vi "Li_New_ADDR_svi.vi"(7 "Op":T1(ring), 8 "error in (no error)":errorcluster, 9 "Addr":i32, 10 "Name":string="FREE") -> (0 "error out":errorcluster, 2 "Size":i32, 3 "Addr":i32)   [LabVIEW 2015]
uses:
  index_cluster.ctl
  C:/Users/Giuseppe/Downloads/LabLinda_ pakage/index_datatype.ctl
  C:/Users/Giuseppe/Downloads/LabLinda_ pakage/index_cluster.ctl
  LIFO.ctl
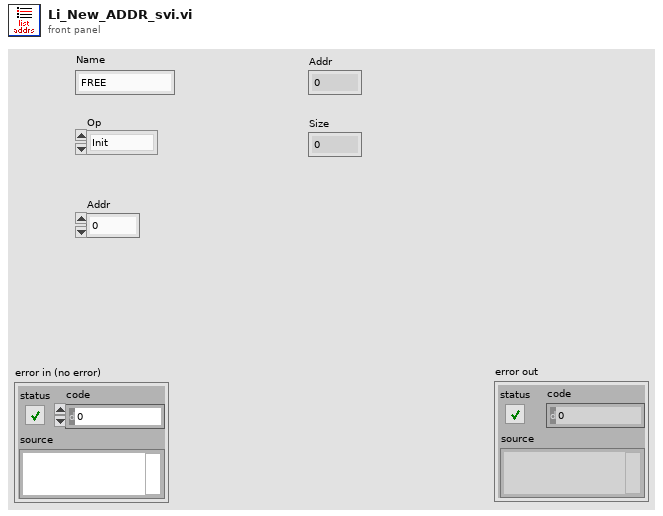
[diagram p1: front panel]
types:
  T1 = enum16{"Init", "Read addr", "Write item", "Cleanup", "Add free", "Query Free"}
  T2 = typedef "index_cluster.ctl" = cluster{"Addr":i32[], "out react vi reference":refnum<vi>, "in react vi reference":refnum<vi>, "rd react vi reference":refnum<vi>, "Read_write_var":refnum<vi>}
  T3 = typedef "LIFO.ctl" = enum16{"INIT", "Push", "Pop", "Query", "BPush"}
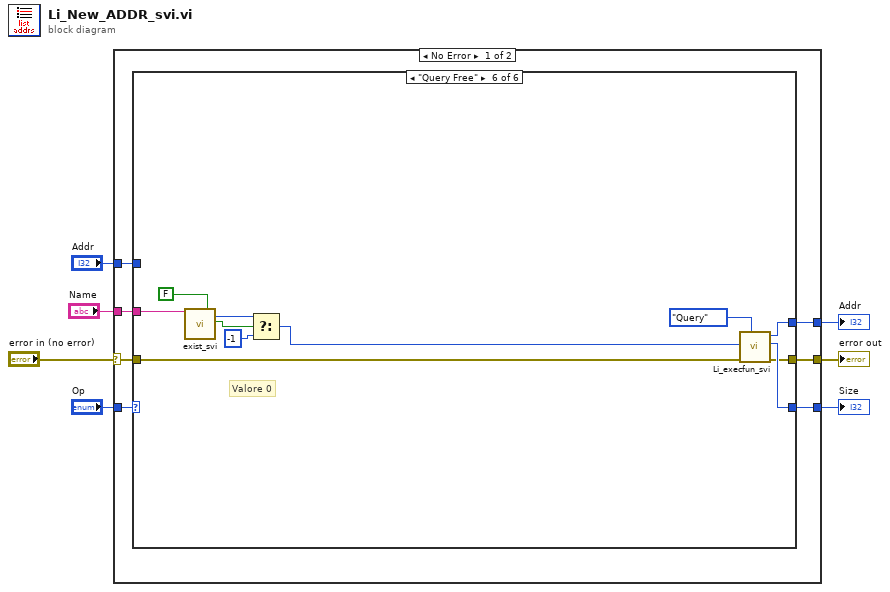
[diagram p0: block diagram]
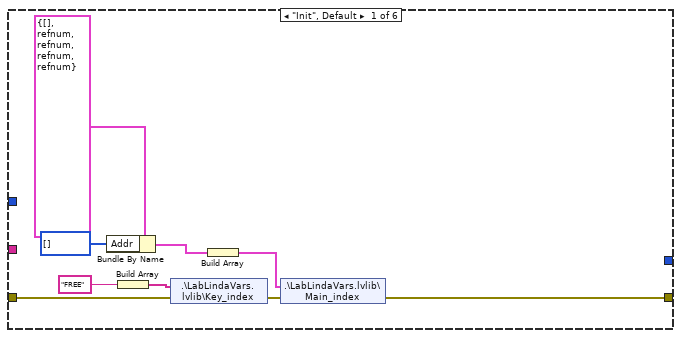
[diagram p2: hidden frame]
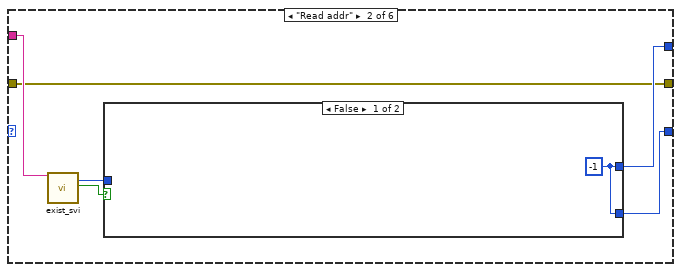
[diagram p3: hidden frame]
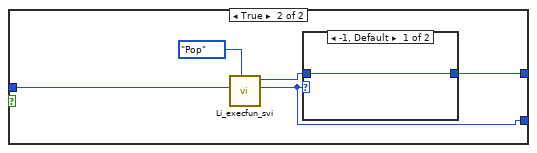
[diagram p4: hidden frame]
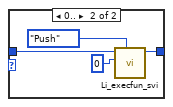
[diagram p5: hidden frame]
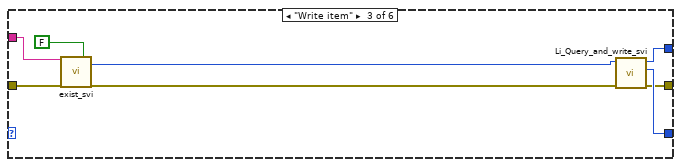
[diagram p6: hidden frame]
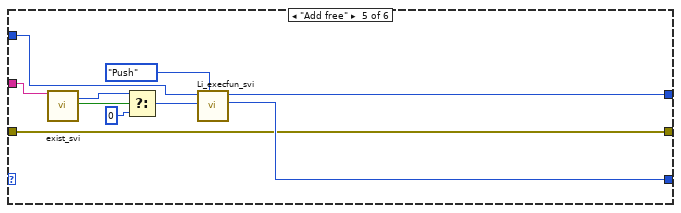
[diagram p8: hidden frame]
diagram:
  n1 = case shown="No Error" "error in (no error)" {
    selector: "error in (no error)" -> [w9 w71]
    tunnel: "Op" -> [w14 _]
    tunnel: "Name" -> [w13 _]
    tunnel: [w12 _] -> w4
    tunnel: [w11 _] -> w3
    tunnel: "Addr" -> [w10 _]
    tunnel: [w8 w71] -> w1
    frame No Error {
      n2 = case shown="\"Query Free\"" w14 {
        tunnel: w13 -> [_ w29 w48 _ w54 w68]
        tunnel: [_ w28 w46 _ w57 w70] -> w12
        tunnel: [_ w27 w47 _ w56 w69] -> w11
        tunnel: w10 -> [_ _ _ _ w59 _]
        tunnel: w9 -> [w18 w26 w43 w49 w55 w61]
        tunnel: [w16 w26 w41 w49 w55 w60] -> w8
        frame "Init", Default {
          n3 = Bundle By Name(cluster=T2 {"Addr"=[], "out react vi reference"=refnum, "in react vi reference"=refnum, "rd react vi reference"=refnum, "Read_write_var"=refnum} ("index_cluster"), "Addr"=i32[] []) -> (w21:T2)
          n4 = Build Array("FREE" ("Name")) -> (w23:string[])
          n5 = shared-variable ".\\LabLindaVars.lvlib\\Key_index"(w23, error in=w18) -> (error out=w17:errorcluster)
          n6 = Build Array(w21) -> (w20:T2[])
          n7 = shared-variable ".\\LabLindaVars.lvlib\\Main_index"(w20, error in=w17) -> (error out=w16:errorcluster)
        }
        frame "Read addr" {
          n8 = call "exist_svi.vi"("Name"=w29) -> ("index of element"=w24:i32, "Exist"=w25:bool)  [unwired: 15 in, 2 out]
          n9 = case shown="False" w25 {
            tunnel: [w30 w35] -> w28
            tunnel: [w30 w33] -> w27
            tunnel: w24 -> [_ w32]
            frame False {
              w30 = -1
            }
            frame True {
              n10 = call "Li_execfun_svi.vi"("OP"=LIFO."Pop", "Key Index"=w32) -> ("Size"=w33:i32, "Addr"=w34:i32)  [unwired: 7 in, 1 out]
              n11 = case shown="-1, Default" w33 {
                tunnel: [w36 w39] -> w35
                tunnel: w34 -> [w36 w38]
                frame -1, Default {
                }
                frame 0.. {
                  n12 = call "Li_execfun_svi.vi"("OP"=enum16{"INIT", "Push", "Pop", "Query"}."Push", "Key Index"=0, "IN"=w38) -> ("Addr"=w39:i32)  [unwired: 6 in, 2 out]
                }
              }
            }
          }
        }
        frame "Write item" {
          n13 = call "exist_svi.vi"("Name"=w48, "error in (no error)"=w43, "Create ?"=FALSE) -> ("index of element"=w44:i32, "error out"=w42:errorcluster)  [unwired: 13 in, 2 out]
          n14 = call "Li_Query_and_write_svi.vi"("error in (no error)"=w42, "Key Index"=w44) -> ("error out"=w41:errorcluster, "Numeric"=w47:i32, "OUT"=w46:i32)  [unwired: 7 in]
        }
        frame "Cleanup" {
        }
        frame "Add free" {
          n15 = call "exist_svi.vi"("Name"=w54) -> ("index of element"=w53:i32, "Exist"=w51:bool)  [unwired: 15 in, 2 out]
          n16 = Select(t=w53, s=w51, f=0) -> (s? t:f=w50:i32)
          n17 = call "Li_execfun_svi.vi"("OP"=enum16{"INIT", "Push", "Pop", "Query"}."Push", "Key Index"=w50, "IN"=w59) -> ("Size"=w56:i32, "Addr"=w57:i32)  [unwired: 6 in, 1 out]
        }
        frame "Query Free" {
          # "Valore 0"
          n18 = call "exist_svi.vi"("Name"=w68, "Create ?"=FALSE) -> ("index of element"=w67:i32, "Exist"=w66:bool)  [unwired: 14 in, 2 out]
          n19 = Select(t=w67, s=w66, f=-1) -> (s? t:f=w64:i32)
          n20 = call "Li_execfun_svi.vi"("OP"=LIFO."Query", "error in (no error)"=w61, "Key Index"=w64) -> ("error out"=w60:errorcluster, "Size"=w69:i32, "Addr"=w70:i32)  [unwired: 6 in]
        }
      }
    }
    frame Error {
    }
  }
  "error out" <- w1
  "Addr" <- w4
  "Size" <- w3
